vi "Initialize.vi"(6 "Version (no version)":string, 7 "API Root":string, 8 "error in (no error)":errorcluster, 9 "Port (protocol specific)":u16, 10 "Base URL":string, 11 "ByteGSAPIBase in":refnum<class "ByteGSAPIBase.lvclass">) -> (0 "error out":errorcluster, 3 "ByteGSAPIBase out":refnum<class "ByteGSAPIBase.lvclass">)   [LabVIEW 2019, in "ByteGSWebAPI.lvlib" / "ByteGSAPIBase.lvclass"]
doc: "Apre una nuova connessione HTTP e setta il content type a \"application/json\""
uses:
  ByteGSAPIBase.lvclass
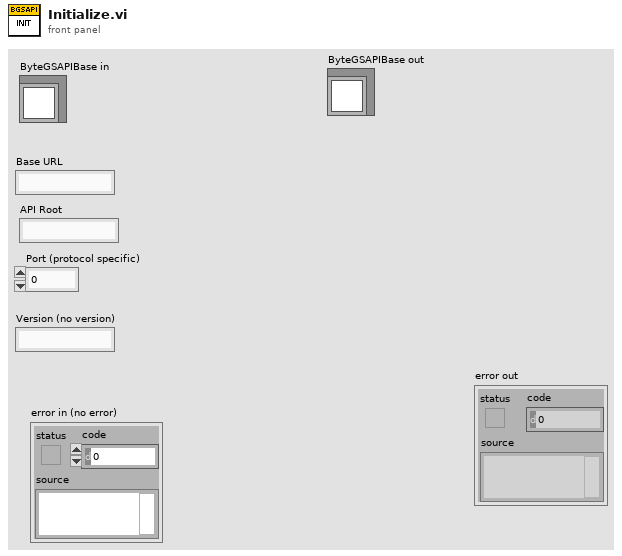
[diagram p1: front panel]
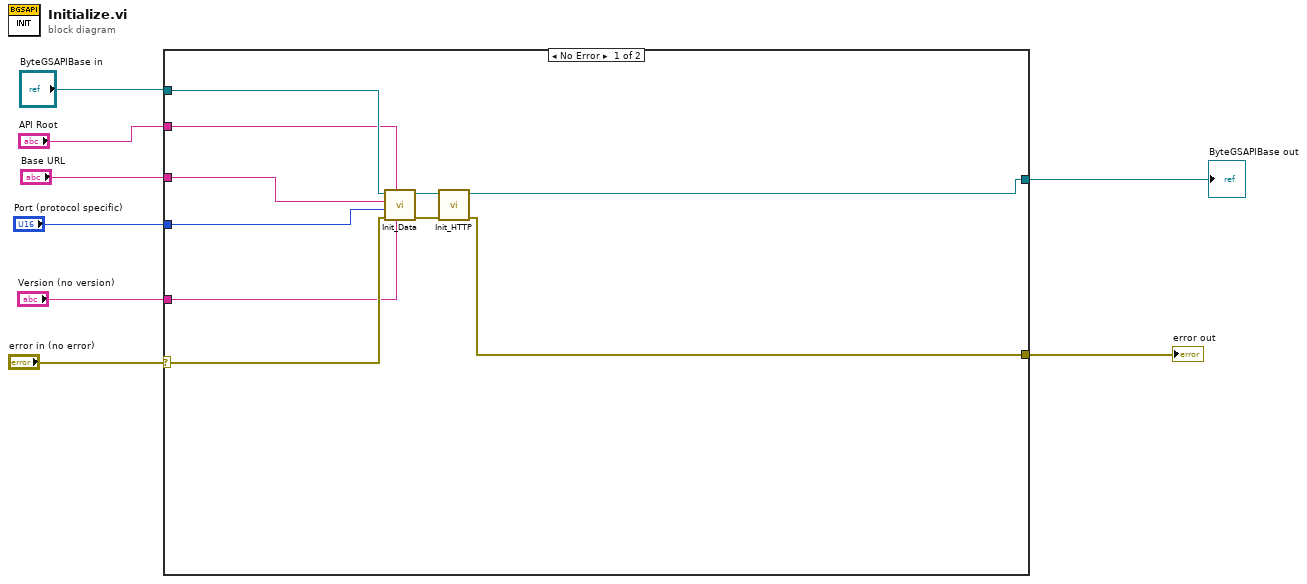
[diagram p0: block diagram]
diagram:
  n1 = case shown="No Error" "error in (no error)" {
    selector: "error in (no error)" -> [w12 w20]
    tunnel: [w10 w20] -> w7
    tunnel: [w9 w19] -> w4
    tunnel: "ByteGSAPIBase in" -> [w16 w19]
    tunnel: "Base URL" -> [w14 _]
    tunnel: "Port (protocol specific)" -> [w13 _]
    tunnel: "Version (no version)" -> [w11 _]
    tunnel: "API Root" -> [w15 _]
    frame No Error {
      n2 = call "Init_Data.vi"("Version (no version)"=w11, "API Root"=w15, "error in (no error)"=w12, "Port (protocol specific)"=w13, "Base URL"=w14, "ByteGSAPIBase in"=w16) -> ("error out"=w17:errorcluster, "ByteGSAPIBase out"=w18:refnum<class "ByteGSAPIBase.lvclass">)  [unwired: 4 in]
      n3 = call "Init_HTTP.vi"("error in (no error)"=w17, "ByteGSAPIBase in"=w18) -> ("error out"=w10:errorcluster, "ByteGSAPIBase out"=w9:refnum<class "ByteGSAPIBase.lvclass">)  [unwired: 8 in]
    }
    frame Error {
    }
  }
  "error out" <- w7
  "ByteGSAPIBase out" <- w4
